vi "속도제어 브레이크PID 연습중.vi"() -> (0 "Platform error out":errorcluster caption="error out")   [LabVIEW 2016]
uses:
  <vilib>/Platform/TimedLoop/XDataNode/timing_clust.ctl
  <vilib>/Platform/TimedLoop/XDataNode/nitl_modes.ctl
  <vilib>/Platform/TimedLoop/XDataNode/wakeup.ctl
  <vilib>/imath/engines/lvmath2/RunTimeEngine/NodeEndStatement/NIMS_NodeEndStatement_Output.vi
  <instcachedir>/0/NIMS_NodeEndStatement_Output_53EC0D466D134D7ABD903AC30B43404B.lvgen/NIMS_NodeEndStatement_Output_53EC0D466D134D7ABD903AC30B43404B_001.vi
  <instcachedir>/0/NIMS_NodeEndStatement_Output_53EC0D466D134D7ABD903AC30B43404B.lvgen/NIMS_NodeEndStatement_Output_53EC0D466D134D7ABD903AC30B43404B_010.vi
  <vilib>/imath/engines/lvmath2/RunTimeEngine/ErrorHandling/NIMS_Finalize Error.vi
  <vilib>/addons/control/pid/pid.llb/PID (DBL).vi
  <vilib>/addons/control/pid/pid.llb/PID Lead-Lag (DBL).vi
  <vilib>/Platform/TimedLoop/XDataNode/XDataNode.xnode
  <vilib>/express/express arith-compare/Formula/XNode/ExpressFormulaBlockNode.xnode
  <vilib>/Platform/TimedLoop/XDataNode/XDNodeRunTimeDep.lvlib
  <vilib>/addons/control/pid/NI_PID_pid.lvlib
panel:
  in  "BRAKE":u16
  in  "SPEED":u16
  in  "PID gains":T1={"proportional gain (Kc)"=1.0, "integral time (Ti, min)"=0.01, "derivative time (Td, min)"=0.0} caption="PID 게인" {"derivative time (Td, min)" format="%#.6g"; "integral time (Ti, min)" format="%#.6g"; "proportional gain (Kc)" format="%#.6g"}
  out "PV Setpoint Output":cluster{"initial PV":dbl, "setpoint":dbl}(graph)={"initial PV"=0.18693112703744846, "setpoint"=0.0}
  in  "정지":bool
  in  "S":dbl=0.5 format="%#_13g"
  in  "Platform error in 2":errorcluster caption="Platform error in"
  in  "Platform Baud rate  2":u32(ring)=115200 items=["Auto Connect"=0, "300"=300, "600"=600, "1200"=1200, "2400"=2400, "4800"=4800, "9600"=9600, "19200"=19200, "38400"=38400, "57600"=57600, "115200"=115200]
  out "Platform Protocol Error":errorcluster
  in  "stop? 3":bool
  out "hex string":string
  out "Encoder_Distance (500ms)":dbl
  in  "stop? 2":bool
  in  "stop?":bool
  in  "Platform error in":errorcluster
  in  "Platform Baud rate":u32(ring)=115200 items=["Auto Connect"=0, "300"=300, "600"=600, "1200"=1200, "2400"=2400, "4800"=4800, "9600"=9600, "19200"=19200, "38400"=38400, "57600"=57600, "115200"=115200]
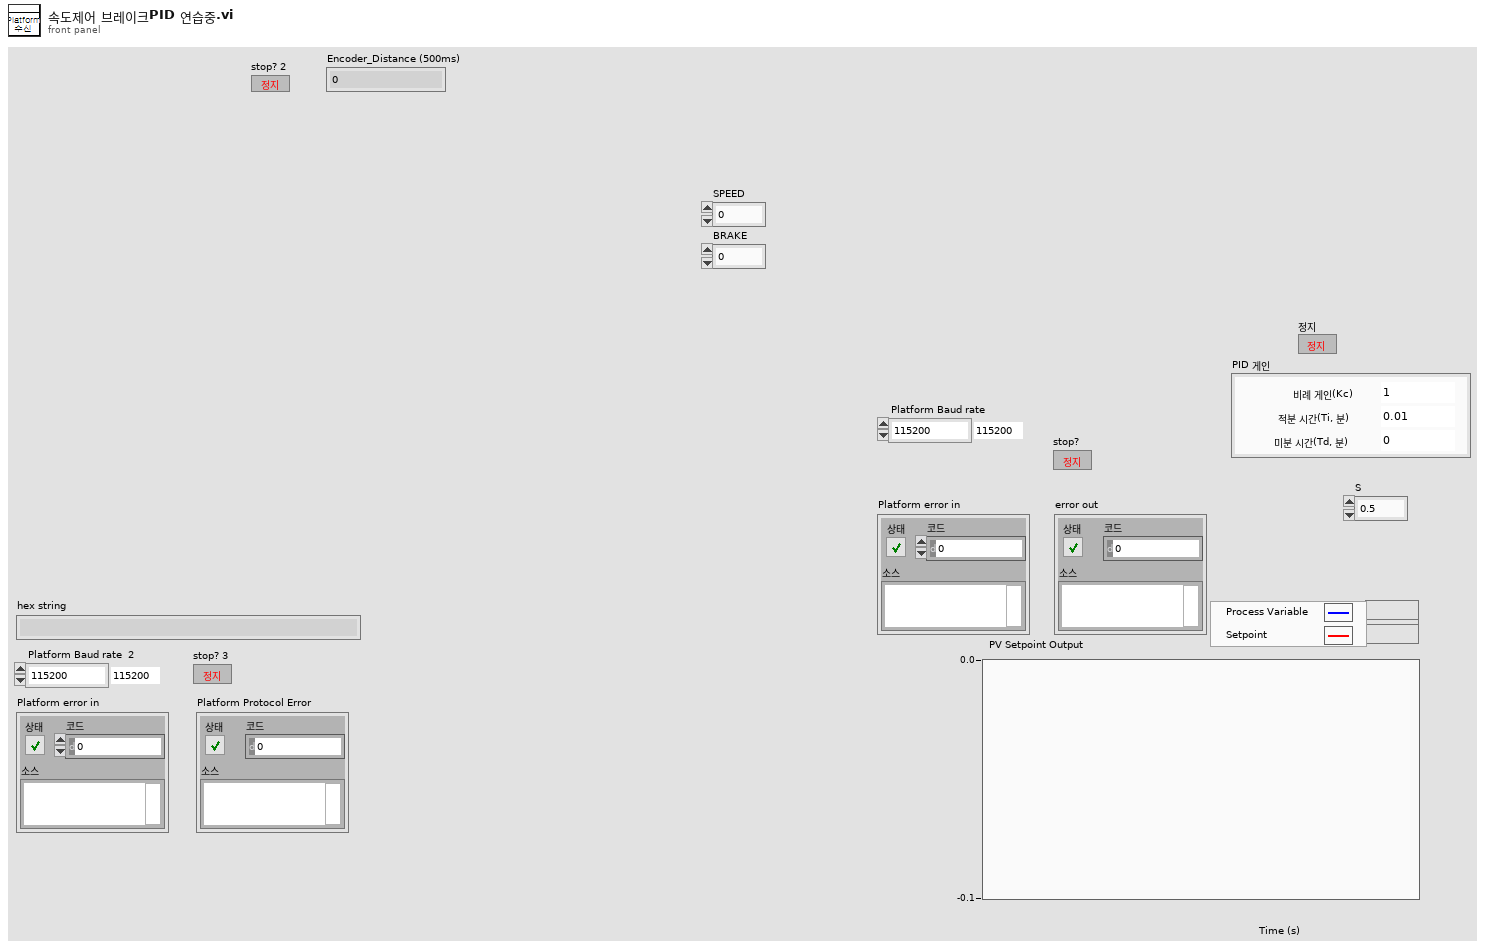
[diagram p1: front panel]
types:
  T1 = cluster{"proportional gain (Kc)":dbl, "integral time (Ti, min)":dbl, "derivative time (Td, min)":dbl}
  T2 = typedef "XDNodeRunTimeDep.lvlib/timing_clust.ctl" = cluster{"Expected End [f-1]":u64, "Actual End [f-1]":u64, "Finished Late? [f-1]":bool, "Expected End [i-1]":u64, "Actual End [i-1]":u64, "Finished Late? [i-1]":bool, "Expected Start [i]":u64, "Actual Start [i]":u64, "Expected Start [f]":u64, "Actual Start [f]":u64, "Source Name":string, "Structure Name":string, "Period":i64, "Deadline":i64, "Offset":i64, "Start":i64, "Priority":i32, "Timeout":i32, "Mode":T3, "Wakeup Reason":T4, "Error":errorcluster, "Source Type":string, "Secondary Source Type":string, "Global End Time":u64, "Global Start Time":u64, "Frame Duration":u64, "Iteration Duration":u64, "Assigned CPU":i32, "I/O Scan Engine Mode":u32}
  T3 = typedef "XDNodeRunTimeDep.lvlib/nitl_modes.ctl" = enum32{"No Change", "Process missed periods, maintain original phase", "Discard missed periods, maintain original phase", "Process missed periods, ignore original phase", "Discard missed periods, ignore original phase"}
  T4 = typedef "XDNodeRunTimeDep.lvlib/wakeup.ctl" = enum32{"Normal", "Aborted", "Asynchronous wakeup", "Timing source error", "Timed loop error", "Timeout"}
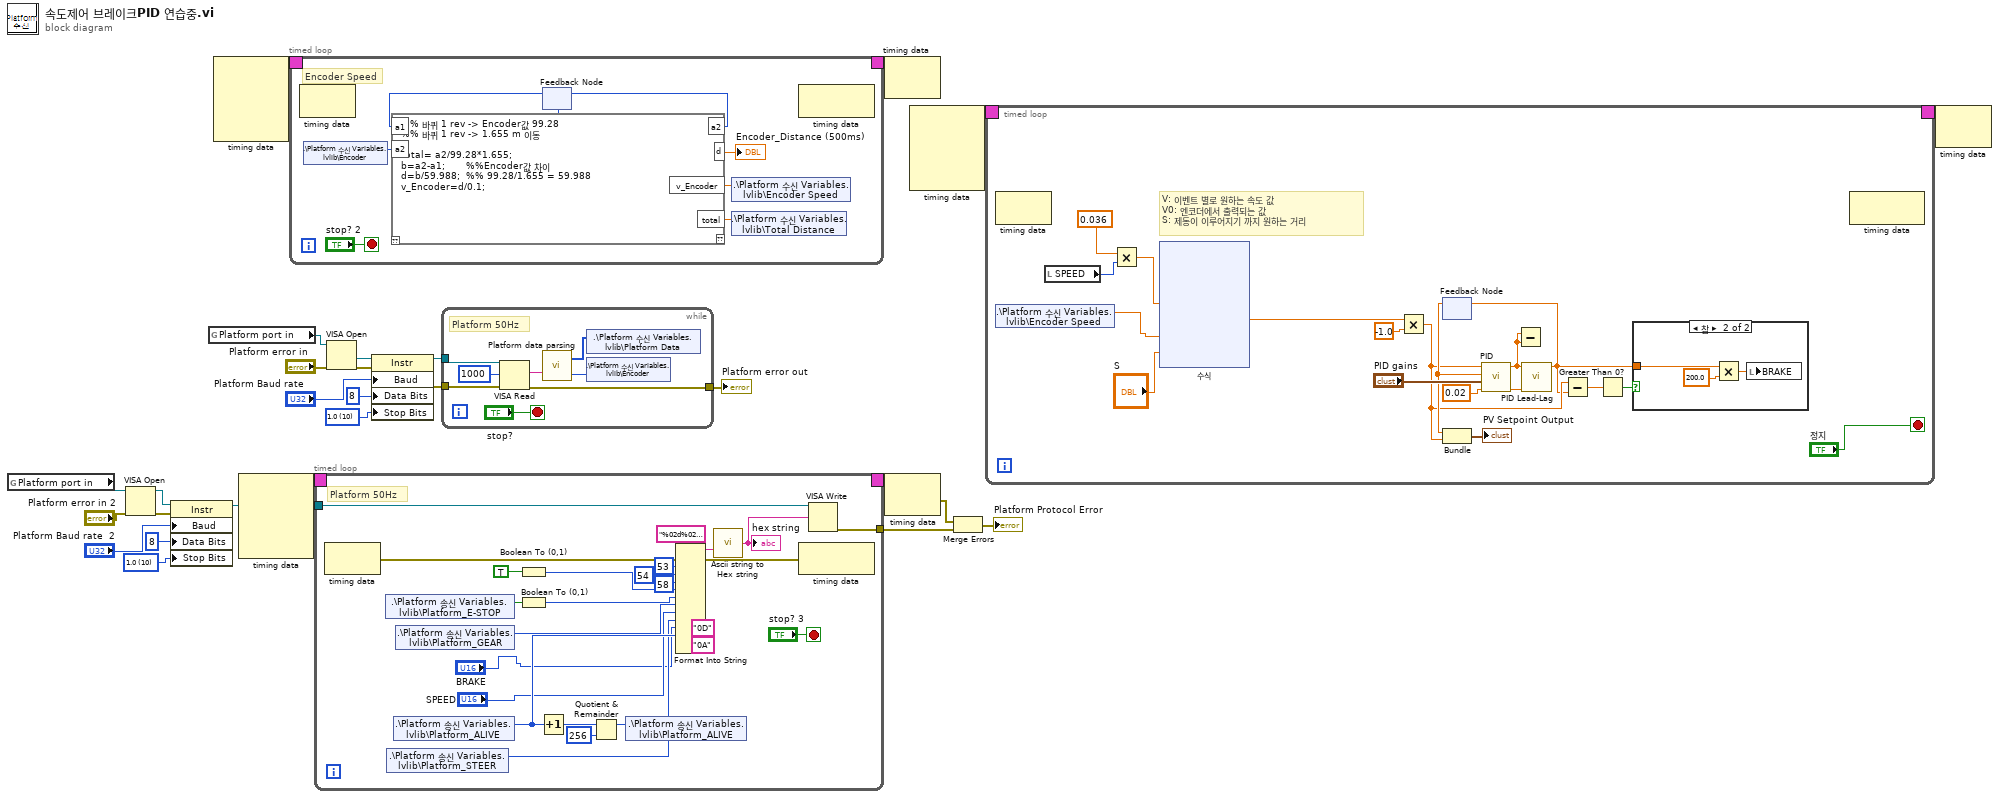
[diagram p0: block diagram]
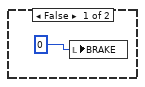
[diagram p2: hidden frame]
diagram:
  w4 = u16 10 items=["1.0"=10, "1.5"=15, "2.0"=20] ("Serial Settings:Stop Bits")
  w26 = u16 10 items=["1.0"=10, "1.5"=15, "2.0"=20] ("Serial Settings:Stop Bits")
  n1 = global read "[GV]_PLATFORM Port NUM.vi" "Platform port in"() -> (w3:refnum<visa-resource-name>)
  n2 = VISA Open(error in (no error)="Platform error in 2", VISA resource name=w3) -> (VISA resource name=w7:refnum<visa-resource-name>, error out=w9:errorcluster)  [unwired: 3 in]
  n3 = property class="Instr"(reference=w7, error in=w9, "Baud"="Platform Baud rate  2", "Data Bits"=u16 8 ("Serial Settings:Data Bits"), "Stop Bits"=w4) -> (reference out=w5:refnum<visa-resource-name>)  [unwired: 1 out]
  n4 = global read "[GV]_PLATFORM Port NUM.vi" "Platform port in"() -> (w18:refnum<visa-resource-name>)
  n5 = node-c288() -> (w17:T2)  [unwired: 4 in]
  n6 = node-c288() -> (w15:T2)  [unwired: 4 in]
  n7 = timed-loop {
    timing: w17 -> [_]
    timing-out: [_] -> w16
    stop <- "stop? 2" stop-if-true
    # "Encoder Speed"
    n8 = node-c288() -> ()  [unwired: 1 in, 1 out]
    n9 = shared-variable ".\\Platform 수신 Variables.lvlib\\Encoder"() -> (w28:i64)  [unwired: 1 in, 1 out]
    n10 = feedback #1(w28) -> (w33:i64)
    n11 = mathscript code="%% 바퀴 1 rev -> Encoder값 99.28\n%% 바퀴 1 rev -> 1.655 m 이동\n\ntotal= a2/99.28*1.655;\nb=a2-a1;       %%Encoder값 차이\nd=b/59.988;  %% 99.28/1.655 = 59.988\nv_Encoder=d/0.1;"("a2"=w28, "a1"=w33) -> ("a2"=w34:i64, "v_Encoder"=w30:dbl, "d"=→"Encoder_Distance (500ms)":dbl, "total"=w29:dbl)  [unwired: 1 in, 1 out]
    n12 = feedback-in #1(w34) -> ()
    n13 = shared-variable ".\\Platform 수신 Variables.lvlib\\Encoder Speed"(w30) -> ()  [unwired: 1 in, 1 out]
    n14 = shared-variable ".\\Platform 수신 Variables.lvlib\\Total Distance"(w29) -> ()  [unwired: 1 in, 1 out]
    n15 = node-c288() -> ()  [unwired: 1 in, 1 out]
  }
  n16 = timed-loop {
    timing: w15 -> [_]
    timing-out: [_] -> w14
    tunnel: [w104] -> w12
    tunnel: w5 -> [w98]
    stop <- "stop? 3" stop-if-true
    # "Platform 50Hz"
    n17 = node-c288() -> (w106:errorcluster)  [unwired: 1 in]
    n18 = shared-variable ".\\Platform 송신 Variables.lvlib\\Platform_E-STOP"() -> (w103:bool)  [unwired: 1 in, 1 out]
    n19 = shared-variable ".\\Platform 송신 Variables.lvlib\\Platform_STEER"() -> (w88:u16)  [unwired: 1 in, 1 out]
    n20 = shared-variable ".\\Platform 송신 Variables.lvlib\\Platform_ALIVE"() -> (w89:u16)  [unwired: 1 in, 1 out]
    n21 = shared-variable ".\\Platform 송신 Variables.lvlib\\Platform_GEAR"() -> (w92:u16)  [unwired: 1 in, 1 out]
    n22 = Boolean To (0,1)(Boolean=TRUE ("Platform_A or M")) -> (0, 1=w94:i16)
    n23 = Boolean To (0,1)(Boolean=w103) -> (0, 1=w93:i16)
    n24 = Increment(x=w89) -> (x+1=w108:u16)
    n25 = Quotient & Remainder(x=w108, y=u16 256) -> (x-y*floor(x/y)=w102:u16)  [unwired: 1 out]
    n26 = shared-variable ".\\Platform 송신 Variables.lvlib\\Platform_ALIVE"(w102) -> ()  [unwired: 1 in, 1 out]
    n27 = Format Into String(format string="%02d%02d%02d%02x%02x%02x%04x%04x%02x%02x%02s%02s" ("포맷 문자열"), error in=w106, u16 53 ("S"), u16 54 ("T"), u16 58 ("X"), w94, w93, w92, "SPEED", w88, "BRAKE", w89, "0D" ("ETX0"), "0A" ("ETX1")) -> (resulting string=w100:string, error out=w105:errorcluster)  [unwired: 1 in]
    n28 = call "Ascii string to Hex string.vi"("ASCII String"=w100) -> ("HEX String"=w99:string)
    "hex string" <- w99
    n29 = node-c288(w105) -> ()  [unwired: 1 out]
    n30 = VISA Write(VISA resource name=w98, write buffer=w99) -> (error out=w104:errorcluster)  [unwired: 1 in, 2 out]
  }
  n31 = VISA Open(error in (no error)="Platform error in", VISA resource name=w18) -> (VISA resource name=w25:refnum<visa-resource-name>, error out=w23:errorcluster)  [unwired: 3 in]
  n32 = property class="Instr"(reference=w25, error in=w23, "Baud"="Platform Baud rate", "Data Bits"=u16 8 ("Serial Settings:Data Bits"), "Stop Bits"=w26) -> (reference out=w21:refnum<visa-resource-name>, error out=w20:errorcluster)
  n33 = while {
    tunnel: w21 -> [w120]
    tunnel: w20 -> [w122]
    tunnel: [w119] -> w19
    stop <- "stop?" stop-if-true
    # "Platform 50Hz"
    n34 = VISA Read(VISA resource name=w120, byte count=u32 1000 ("바이트 카운트"), error in (no error)=w122) -> (read buffer=w117:string, error out=w119:errorcluster)  [unwired: 2 out]
    n35 = call "Platform data parsing.vi"("Platform Data"=w117) -> ("Encoder"=w116:i64, "Platform Data Array"=w115:i64[])  [unwired: 2 in]
    n36 = shared-variable ".\\Platform 수신 Variables.lvlib\\Platform Data"(w115) -> ()  [unwired: 1 in, 1 out]
    n37 = shared-variable ".\\Platform 수신 Variables.lvlib\\Encoder"(w116) -> ()  [unwired: 1 in, 1 out]
  }
  "Platform error out" <- w19
  n38 = node-c288(w16) -> ()  [unwired: 1 out]
  n39 = node-c288(w14) -> (w13:errorcluster)
  n40 = node-c288() -> (w2:T2)  [unwired: 4 in]
  n41 = Merge Errors(w13, w12) -> (→"Platform Protocol Error":errorcluster)
  n42 = timed-loop {
    timing: w2 -> [_]
    timing-out: [_] -> w1
    stop <- "정지" stop-if-true
    # "V: 이벤트 별로 원하는 속도 값\nV0: 엔코더에서 출력되는 값\nS: 제동이 이루어지기 까지 원하는 거리"
    n43 = node-c288() -> ()  [unwired: 1 in, 1 out]
    n44 = shared-variable ".\\Platform 수신 Variables.lvlib\\Encoder Speed"() -> (w126:dbl)  [unwired: 1 in, 1 out]
    n45 = local read "SPEED"() -> (w125:u16)
    n46 = Multiply(x=0.036, y=w125) -> (x*y=w124:dbl)
    n47 = xnode "수식"("V"=w124, "V0"=w126, "S"="S") -> ("결과"=w131:dbl)  [unwired: 1 in, 1 out]
    n48 = Multiply(x=w131, y=-1.0) -> (x*y=w129:dbl)
    n49 = feedback #2() -> (w137:dbl)  [unwired: 1 in]
    n50 = Bundle("output"=w137, w129) -> (→"PV Setpoint Output":cluster{"output":dbl, dbl})  [unwired: 1 in]
    n51 = call-poly <vilib>:"PID.vi"("dt (s)"=0.02, "PID gains"="PID gains", "process variable"=w137, "setpoint"=w129) -> ("dt out (s)"=w135:dbl, "output"=w134:dbl)  [unwired: 6 in]
    n52 = Subtract(x=w134, y=w134) -> ()  [unwired: 1 out]
    n53 = call-poly <vilib>:"PID Lead-Lag.vi"("dt (s)"=w135, "input"=w134) -> ("output"=w128:dbl)  [unwired: 6 in, 1 out]
    n54 = feedback-in #2(w128) -> ()
    n55 = Subtract(x=w129, y=w128) -> (x-y=w127:dbl)
    n56 = Greater Than 0?(x=w127) -> (x > 0?=w130:bool)
    n57 = case shown="참" w130 {
      tunnel: w128 -> [_ w156]
      frame False {
        n58 = local write "BRAKE"(i16 0 ("brake")) -> ()
      }
      frame True {
        n59 = Multiply(x=w156, y=200.0) -> (x*y=w155:dbl)
        n60 = local write "BRAKE"(w155) -> ()
      }
    }
    n61 = node-c288() -> ()  [unwired: 1 in, 1 out]
  }
  n62 = node-c288(w1) -> ()  [unwired: 1 out]
